vi "ModeArmScoring.vi"() -> (0 "Scoring Position":T1(ring))   [LabVIEW 2020]
doc: "Determines the scoring mode and outputs the goal scoring position based on the manipulator commands and the sensed game piece held by the gripper."
uses:
  GlobalDriverStationCommands.vi
  GlobalGripper.vi
  45ffc62e-e0ac-4f04-9749-09a6b17a6dc4.vi
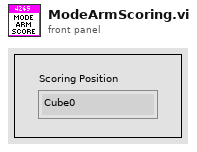
[diagram p1: front panel]
types:
  T1 = enum16{"Cube0", "Cube1", "Cube2", "Cone0", "Cone1", "Cone2"}
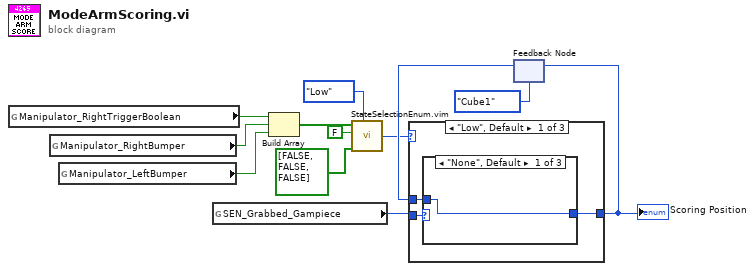
[diagram p0: block diagram]
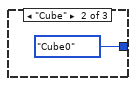
[diagram p2: hidden frame]
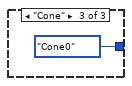
[diagram p3: hidden frame]
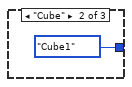
[diagram p5: hidden frame]
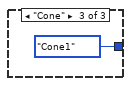
[diagram p6: hidden frame]
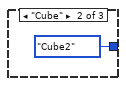
[diagram p8: hidden frame]
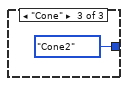
[diagram p9: hidden frame]
diagram:
  n1 = global read "GlobalDriverStationCommands.vi" "Manipulator_RightTriggerBoolean"() -> (w10:bool)
  n2 = global read "GlobalDriverStationCommands.vi" "Manipulator_RightBumper"() -> (w9:bool)
  n3 = global read "GlobalDriverStationCommands.vi" "Manipulator_LeftBumper"() -> (w8:bool)
  n4 = global read "GlobalGripper.vi" "SEN_Grabbed_Gampiece"() -> (w12:enum16{"None", "Cube", "Cone"})
  n5 = Build Array(w10, w9, w8) -> (w7:bool[])
  n6 = call "StateSelectionEnum.vim"("Enum Def"=enum16{"Low", "Mid", "High"}."Low", "Disallowed States"=bool[] [FALSE, FALSE, FALSE], "Enable Edge Trigger"=FALSE, "State Triggers"=w7) -> ("Selected State"=w4:enum16{"Low", "Mid", "High"})  [unwired: 1 in, 1 out]
  n7 = feedback #1(T1."Cube1" ("Scoring Position")) -> (w11:T1)
  n8 = case shown="\"Low\", Default" w4 {
    tunnel: w12 -> [w15 w21 w26]
    tunnel: [w13 w19 w25] -> w1
    tunnel: w11 -> [w14 w20 w27]
    frame "Low", Default {
      n9 = case shown="\"None\", Default" w15 {
        tunnel: [w16 T1."Cube0" ("Scoring Position") T1."Cone0" ("Scoring Position")] -> w13
        tunnel: w14 -> [w16 _ _]
        frame "None", Default {
        }
        frame "Cube" {
        }
        frame "Cone" {
        }
      }
    }
    frame "Mid" {
      n10 = case shown="\"None\", Default" w21 {
        tunnel: [w22 T1."Cube1" ("Scoring Position") T1."Cone1" ("Scoring Position")] -> w19
        tunnel: w20 -> [w22 _ _]
        frame "None", Default {
        }
        frame "Cube" {
        }
        frame "Cone" {
        }
      }
    }
    frame "High" {
      n11 = case shown="\"None\", Default" w26 {
        tunnel: [w28 T1."Cube2" ("Scoring Position") T1."Cone2" ("Scoring Position")] -> w25
        tunnel: w27 -> [w28 _ _]
        frame "None", Default {
        }
        frame "Cube" {
        }
        frame "Cone" {
        }
      }
    }
  }
  "Scoring Position" <- w1
  n12 = feedback-in #1(w1) -> ()
